vi "Easy VI Analysis.vi"() -> ()   [LabVIEW 2023]
doc: "This example uses the \"Easy\" VI Analyzer VIs to perform an analysis based on the settings in a CFG file that was created through the VI Analyzer user interface. Once the analysis performed by \"VIAn Easy Analyze.vi\" is complete, the \"VIAn Easy Report.vi\" saves the analysis results to an HTML report."
uses:
  <vilib>/Platform/browser.llb/Open URL in Default Browser (path).vi
  <vilib>/addons/analyzer/NI_VIAnalyzerTKVIs.lvlib
panel:
  out "Total Analysis Time":dbl format="%<%M min, %S%2u sec>t"
  out "% Failed":dbl format="%.1f%%"
  out "% Passed":dbl format="%.1f%%"
  # "Overview: Demonstrates the use of the \"Easy\" VI Analyzer VIs to perform a programmatic analysis.\nRequirements: VI Analyzer Toolkit\nInstructions:\nRun the VI."
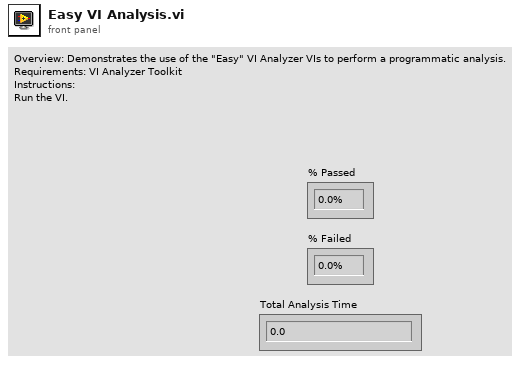
[diagram p1: front panel]
types:
  T1 = typedef "VIAnCtl Results.ctl" = cluster{"Test Name":string, "Results Data":T2[], "Status":T3, "Exceed Max Fails?":bool}
  T2 = typedef "VIAnCtl ResultsData (index).ctl" = cluster{"Result Message":string, "Ref Index":i32}
  T3 = typedef "VIAnCtl ResultStatus.ctl" = enum16{"Pass", "Fail", "Skipped", "VI not loadable", "Test not loadable", "Test not runnable", "Test error out"}
  T4 = typedef "VIAnRes Parsed Results Data (by VI).ctl" = cluster{"VI Path":path, "Pass":cluster{"row":i32, "column":i32}[], "Fail":cluster{"row":i32, "column":i32}[], "Skipped":cluster{"row":i32, "column":i32}[], "VI not loadable":cluster{"row":i32, "column":i32}[], "Test not loadable":cluster{"row":i32, "column":i32}[], "Test not runnable":cluster{"row":i32, "column":i32}[], "Test error out":cluster{"row":i32, "column":i32}[]}
  T5 = typedef "VIAnRes Parsed Results Data (by Test).ctl" = cluster{"Test Name":string, "Pass":cluster{"VI Path":path, "index":cluster{"row":i32, "column":i32}}[], "Fail":cluster{"VI Path":path, "index":cluster{"row":i32, "column":i32}}[], "Skipped":cluster{"VI Path":path, "index":cluster{"row":i32, "column":i32}}[]}
  T6 = typedef "VIAnCtl Test Config Data.ctl" = cluster{"Test Name":string, "Config Ref":refnum<vi>, "Ref Valid?":bool, "Test Ranking":T7, "Max Failures":u32, "Test Path":path, "Control Values":T8[], "Selected?":bool}
  T7 = typedef "VIAnCtl TestRanking.ctl" = u16
  T8 = typedef "VIAnCtl Config Control Value.ctl" = cluster{"Control Name":string, "Control Value":variant}
  T9 = cluster{"Raw Results":T1[][], "Parsed Results Data (by VI)":T4[], "Parsed Results Data (by Test)":T5[], "Summary Statistics":cluster{"Passed Tests":i32, "Failed Tests":i32, "Skipped Tests":i32, "VIs not loadable":i32, "Tests not loadable":i32, "Tests not runnable":i32, "Test error out":i32, "Start Time":u32, "Total Time (s)":dbl}, "Test Config Data":T6[]}
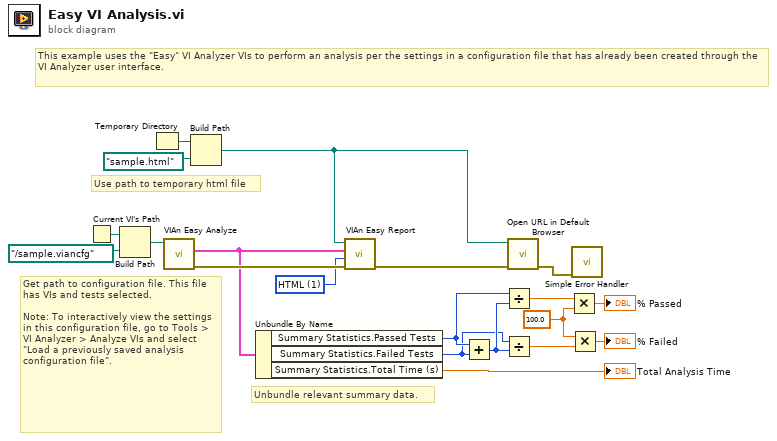
[diagram p0: block diagram]
diagram:
  w5 = 100.0
  w16 = u16 1 items=["ASCII", "HTML", "RSL File"] ("Report Save Type (ASCII)")
  # "Use path to temporary html file"
  # "This example uses the \"Easy\" VI Analyzer VIs to perform an analysis per the settings in a configuration file that has already been created through the VI Analyzer user interface."
  # "Get path to configuration file. This file has VIs and tests selected.\n \nNote: To interactively view the settings in this configuration file, go to Tools > VI Analyzer > Analyze VIs and select \"Load a previously saved analysis configuration file\"."
  # "Unbundle relevant summary data."
  n1 = Current VI's Path() -> (path=w19:path)
  n2 = Build Path(base path=w19, name or relative path=path "../sample.viancfg" ("path")) -> (appended path=w17:path)
  n3 = Temporary Directory() -> (w13:path)
  n4 = call <vilib>:"VIAn Easy Analyze.vi"("Analysis Target"=w17) -> ("error out"=w20:errorcluster, "Analysis Results"=w15:T9)  [unwired: 2 in, 7 out]
  n5 = Build Path(base path=w13, name or relative path=path "sample.html" ("path")) -> (appended path=w3:path)
  n6 = Unbundle By Name(w15) -> ("Summary Statistics.Passed Tests"=w10:i32, "Summary Statistics.Failed Tests"=w4:i32, "Summary Statistics.Total Time (s)"=→"Total Analysis Time":dbl)
  n7 = call <vilib>:"VIAn Easy Report.vi"("error in (no error)"=w20, "Report Save Type (ASCII)"=w16, "Analysis Results"=w15, "Report Save Path"=w3) -> ("error out"=w2:errorcluster)  [unwired: 3 in, 4 out]
  n8 = Add(x=w10, y=w4) -> (x+y=w11:i32)
  n9 = Divide(x=w10, y=w11) -> (x/y=w9:dbl)
  n10 = Divide(x=w4, y=w11) -> (x/y=w8:dbl)
  n11 = call-poly <vilib>:"Open URL in Default Browser.vi"("error in (no error)"=w2, "path"=w3) -> ("error out"=w1:errorcluster)  [unwired: 5 out]
  n12 = Multiply(x=w9, y=w5) -> (x*y=→"% Passed":dbl)
  n13 = Multiply(x=w5, y=w8) -> (x*y=→"% Failed":dbl)
  n14 = call <vilib>:"Simple Error Handler.vi"("error in (no error)"=w1) -> ()  [unwired: 4 in, 5 out]
